vi "read build spec name.vi"(11 "Builders in":refnum<class "Builder.lvclass">) -> (2 "build spec name":string)   [LabVIEW 2024, in "Builder.lvclass"]
uses:
  Builder.lvclass
  Builder.lvclass/Builder.ctl
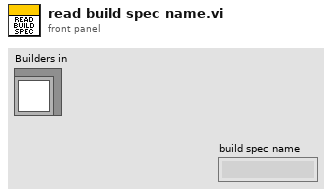
[diagram p1: front panel]
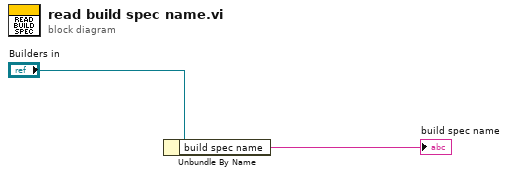
[diagram p0: block diagram]
diagram:
  n1 = Unbundle By Name("Builders in") -> ("build spec name"=→"build spec name":string)
